vi "Palindromic Word Detector with monitor.vi"() -> ()   [LabVIEW 2017]
panel:
  out "Palindrome?":bool
  in  "Word":string
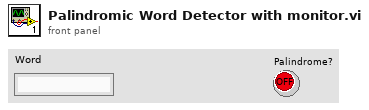
[diagram p1: front panel]
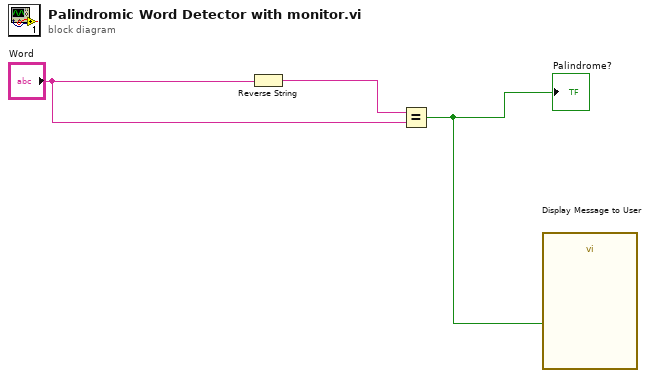
[diagram p0: block diagram]
diagram:
  n1 = Reverse String(1:"Word") -> (0:w2:string)
  n2 = Equal?(x=w2, y="Word") -> (x = y?=w1:bool)
  "Palindrome?" <- w1
  n3 = call "Display Message to User"("Enable"=w1) -> ()  [unwired: 9 in, 2 out]
